vi "lib_QMH_Get Show Diagram on Init.vi"(8 "error in (no error)":errorcluster caption="错误输入（无错误）", 11 "Module Admin in":refnum<class "lib_QMH_Module_Admin.lvclass">) -> (0 "error out":errorcluster caption="错误输出", 2 "Show Diagram on Init":bool, 3 "Module_Admin out":refnum<class "lib_QMH_Module_Admin.lvclass">)   [LabVIEW 2018, in "lib_QMH_Module_Admin.lvclass"]
uses:
  lib_QMH_Module_Admin.lvclass
  lib_QMH_Module_Admin.lvclass/lib_QMH_Module_Admin.ctl
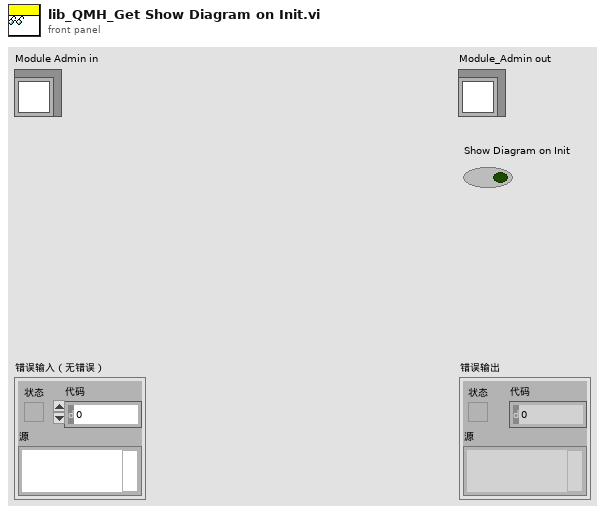
[diagram p1: front panel]
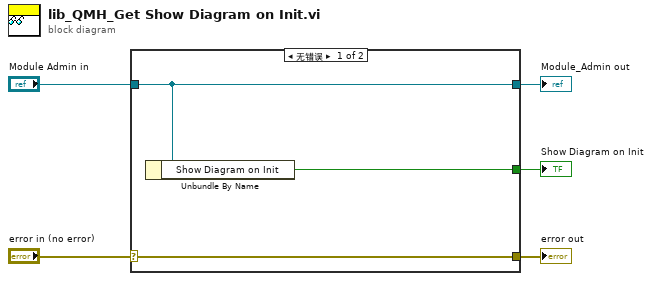
[diagram p0: block diagram]
diagram:
  n1 = case shown="无错误" "error in (no error)" {
    selector: "error in (no error)" -> [w8 w9]
    tunnel: [w8 w9] -> w4
    tunnel: [w7 w10] -> w2
    tunnel: "Module Admin in" -> [w7 w10]
    tunnel: [w6 _] -> w1
    frame No Error {
      n2 = Unbundle By Name(w7) -> ("Show Diagram on Init"=w6:bool)
    }
    frame Error {
    }
  }
  "error out" <- w4
  "Module_Admin out" <- w2
  "Show Diagram on Init" <- w1
